vi "Update Service Completion.vi"(0 "File Data Manager in":refnum<class "File Data Manager.lvclass">, 5 "Service ID":string[](array[string]), 11 "error in (no error)":errorcluster) -> (4 "File Data Manager out":refnum<class "File Data Manager.lvclass">, 15 "error out":errorcluster)   [LabVIEW 2023, in "File Data Manager.lvlib" / "File Data Manager.lvclass"]
uses:
  File Data Manager.lvclass
  File Data Manager.lvclass/File Data Manager.ctl
  <vilib>/Utility/miscctls.llb/LVMapReplaceAction.ctl
  <vilib>/ActorFramework/Actor/Actor.lvclass
  Central Data Manager/Central Data Manager Messages/Refresh Rooms Status Msg/Refresh Rooms Status Msg.lvclass
  Room Service Types/Room Service Base/Room Service Base.lvclass
  C:/Users/bhaghyaraj/Trainings/NI Actor Framework/SDLC/Central Data Manager/Central Data Manager/Central Data Manager.lvclass
  C:/Users/bhaghyaraj/Trainings/NI Actor Framework/SDLC/Model Base/Model Base/Model Base.lvclass
  C:/Program Files/National Instruments/LabVIEW 2023/vi.lib/ActorFramework/Actor/Actor.lvclass
  C:/Users/bhaghyaraj/Trainings/NI Actor Framework/SDLC/Interfaces/Model Base/Incoming Model Base Interface.lvclass
  C:/Users/bhaghyaraj/Trainings/NI Actor Framework/SDLC/File Data Manager/File Data Manager/File Data Manager.lvclass
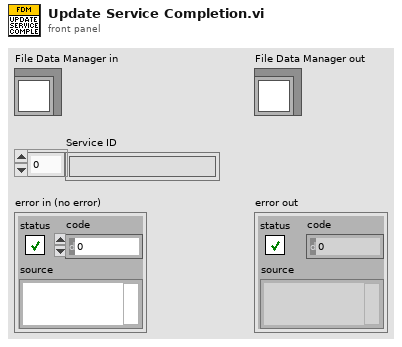
[diagram p1: front panel]
types:
  T1 = map{string, map{string, refnum<class "Room Service Base.lvclass">}}
  T2 = map{string, refnum<class "Room Service Base.lvclass">}
  T3 = typedef "LVMapReplaceAction.ctl" = enum32{"Modify Entry only if found", "Add or Modify Entry", "Delete Entry"}
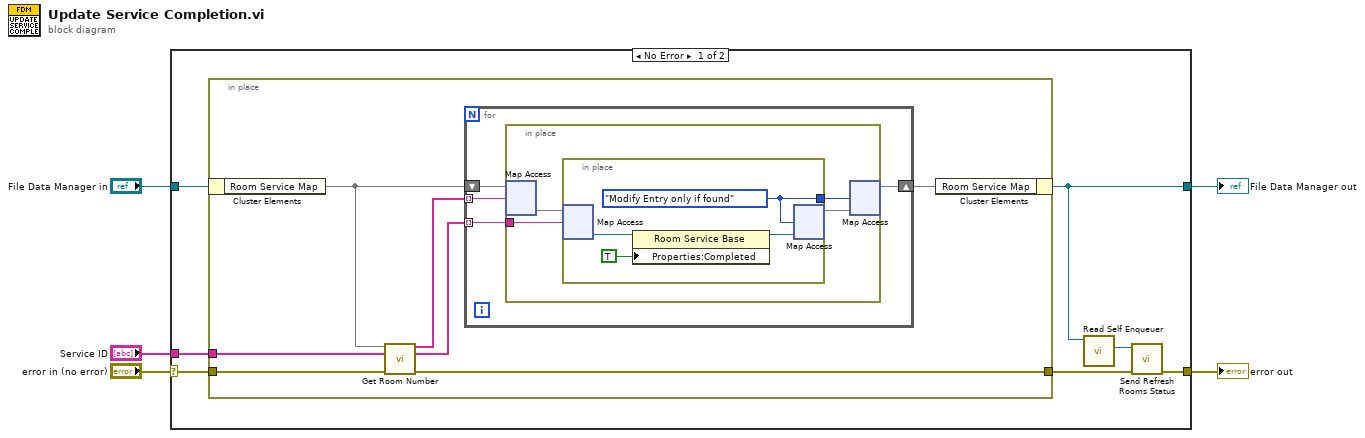
[diagram p0: block diagram]
diagram:
  n1 = case shown="No Error" "error in (no error)" {
    selector: "error in (no error)" -> [w11 w32]
    tunnel: [w7 w32] -> w4
    tunnel: "File Data Manager in" -> [w9 w33]
    tunnel: [w8 w33] -> w2
    tunnel: "Service ID" -> [w12 _]
    frame No Error {
      n2 = in-place {
        in-place-border: w12 -> [w15]
        in-place-border: w11 -> [w18]
        in-place-border: [w17] -> w10
        n3 = in-place-cluster #1(w9) -> ("Room Service Map"=w16:T1)
        n4 = call "Get Room Number.vi"("Room Service Map"=w16, "Service ID"=w15, "error in (no error)"=w18) -> ("Room Number"=w14:string[], "Service ID"=w13:string[], "error out"=w17:errorcluster)  [unwired: 10 in]
        n5 = for {
          shift-right: [w22] -> w19
          shift-left: w16 -> [w23]
          tunnel: w14 -> [w21] mode=indexing
          tunnel: w13 -> [w20] mode=indexing
          n6 = in-place {
            in-place-border: w20 -> [w25]
            n7 = in-place-map #2(w23, w21) -> (w27:T2)  [unwired: 1 in, 1 out]
            n8 = in-place {
              in-place-border: [w29] -> w24
              w29 = LVMapReplaceAction."Modify Entry only if found" ("action")
              n9 = in-place-map #3(w27, w25) -> (w28:refnum<class "Room Service Base.lvclass">)  [unwired: 1 in, 1 out]
              n10 = property class="Room Service Base"(reference=w28, "Properties:Completed"=TRUE ("Completed")) -> (reference out=w31:refnum<class "Room Service Base.lvclass">)  [unwired: 1 in, 1 out]
              n11 = in-place-map #3(w31, w29) -> (w26:T2)  [unwired: 2 out]
            }
            n12 = in-place-map #2(w26, w24) -> (w22:T1)  [unwired: 2 out]
          }
        }
        n13 = in-place-cluster #1("Room Service Map"=w19) -> (w8:refnum<class "File Data Manager.lvclass">)
      }
      n14 = call <vilib>:"Read Self Enqueuer.vi"("Actor"=w8) -> ("Self Enqueuer"=w6:refnum<class "Message Enqueuer.lvclass">)  [unwired: 10 in]
      n15 = call "Send Refresh Rooms Status.vi"("error in (no error)"=w10, "Message Enqueuer"=w6) -> ("error out"=w7:errorcluster)  [unwired: 8 in, 1 out]
    }
    frame Error {
    }
  }
  "error out" <- w4
  "File Data Manager out" <- w2
